vi "Design and Apply Savitzky-Golay Filter.vi"() -> ()   [LabVIEW 2020]
doc: "This example demonstrates how to use the Savitzky-Golay Filter Coefficients.vi to design a Savitzky-Golay filter and use it to smooth a noisy signal."
uses:
  <vilib>/Analysis/baseanly.llb/Real Dot Product.vi
  <vilib>/Analysis/baseanly.llb/A x Vector.vi
  <vilib>/Analysis/NI_AALBase.lvlib
panel:
  in  "seed":i32=-1
  in  "Stop":bool
  out "Graph":dbl[][](graph)
  in  "samples":i32=300
  in  "polynomial order":i32(slide)=8 scale=0.0..20.0
  in  "side points":i32(slide)=12 scale=0.0..50.0
  # "Overview: Demonstrates how to use the Savitzky-Golay Filter Coefficients VI to design a Savitzky-Golay filter that smoothes a noisy signal.\nRequirements: LabVIEW Full Development System.\nInstructions:\n1. Run the VI to see the noisy and smoothed signals.\n2. Modify the side points and polynomial order.\n3. Change seed to a positive number to generate the same noisy signal.\n4. Click Stop to stop the VI."
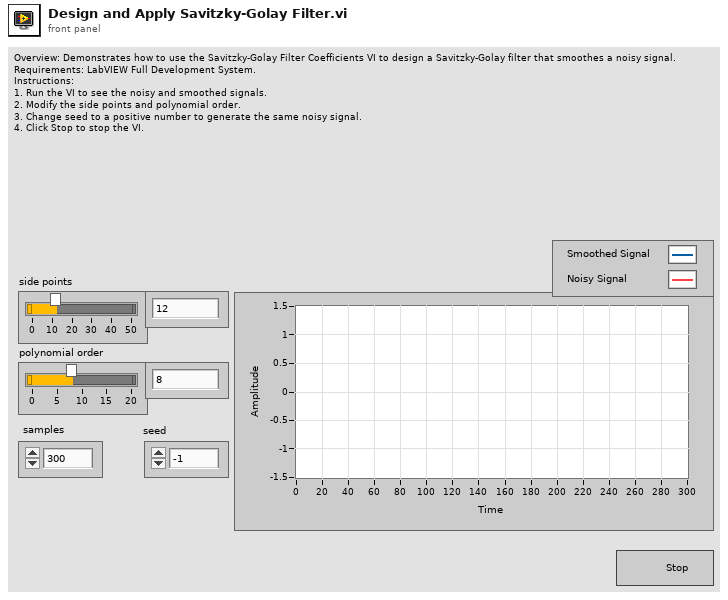
[diagram p1: front panel]
types:
  T1 = typedef "NI_Matrix.lvlib/RealMatrix.ctl" = dbl[][]
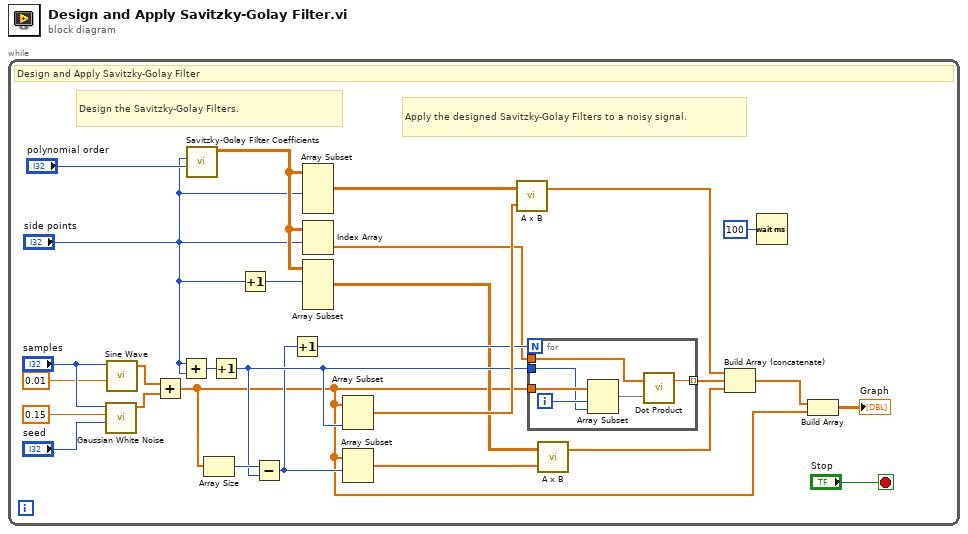
[diagram p0: block diagram]
diagram:
  n1 = while {
    stop <- "Stop" stop-if-true
    # "Apply the designed Savitzky-Golay Filters to a noisy signal."
    # "Design the Savitzky-Golay Filters."
    # "Design and Apply Savitzky-Golay Filter"
    n2 = call <vilib>:"Gaussian White Noise.vi"("seed"="seed", "standard deviation"=0.15, "samples"="samples") -> ("Gaussian noise pattern"=w10:dbl[])  [unwired: 7 in, 1 out]
    n3 = call <vilib>:"Sine Wave.vi"("samples"="samples", "frequency"=0.01 ("f")) -> ("sine wave"=w11:dbl[])  [unwired: 3 in, 2 out]
    n4 = Add(x=w11, y=w10) -> (x+y=w1:dbl[])
    n5 = Add(x="side points", y="side points") -> (x+y=w26:i32)
    n6 = call <vilib>:"Savitzky-Golay Filter Coefficients.vi"("polynomial order"="polynomial order", "side points"="side points") -> ("Savitzky-Golay Filters"=w19:T1)  [unwired: 7 in, 2 out]
    n7 = Array Size(array=w1) -> (size(s)=w24:i32)
    n8 = Increment(x=w26) -> (x+1=w23:i32)
    n9 = Increment(x="side points") -> (x+1=w27:i32)
    n10 = Subtract(x=w24, y=w23) -> (x-y=w22:i32)
    n11 = Increment(x=w22) -> (x+1=w21:i32)
    n12 = Array Subset(array=w19, length (row)="side points") -> (w28:T1)  [unwired: 3 in]
    n13 = Index Array(array=w19, index (row)="side points") -> (element=w20:dbl[])  [unwired: 1 in]
    n14 = Array Subset(array=w19, index (row)=w27) -> (w18:T1)  [unwired: 3 in]
    n15 = Array Subset(array=w1, length=w23) -> (w25:dbl[])  [unwired: 1 in]
    n16 = Array Subset(array=w1, index=w22) -> (w17:dbl[])  [unwired: 1 in]
    n17 = call-poly <vilib>:"A x B.vi"("Vector"=w25, "A"=w28) -> ("A x Vector"=w16:dbl[])  [unwired: 1 out]
    n18 = for {
      N: w21 -> [_]
      tunnel: w1 -> [w34]
      tunnel: w23 -> [w32]
      tunnel: w20 -> [w31]
      tunnel: [w29] -> w15 mode=indexing
      i -> [w33]
      n19 = Array Subset(array=w34, index=w33, length=w32) -> (w30:dbl[])
      n20 = call-poly <vilib>:"Dot Product.vi"("Y Vector"=w30, "X Vector"=w31) -> ("X * Y"=w29:dbl)  [unwired: 1 out]
    }
    n21 = call-poly <vilib>:"A x B.vi"("Vector"=w17, "A"=w18) -> ("A x Vector"=w14:dbl[])  [unwired: 1 out]
    n22 = Build Array (concatenate)(w16, w15, w14) -> (w9:dbl[])
    n23 = Wait (ms)(milliseconds to wait=u32 100) -> ()  [unwired: 1 out]
    n24 = Build Array(w9, w1) -> (→"Graph":dbl[][])
  }
